vi "Reference Generation.vi"(8 "error in (no error)":errorcluster, 11 "VI in":refnum<vi>) -> (0 "error out":errorcluster, 3 "User Events Reference":refnum<event-registration>)   [LabVIEW 2014, in "User Module.lvlib"]
uses:
  User Module.lvlib
  User Event/User Event Action.ctl
  Queue FGV.ctl
  Message.ctl
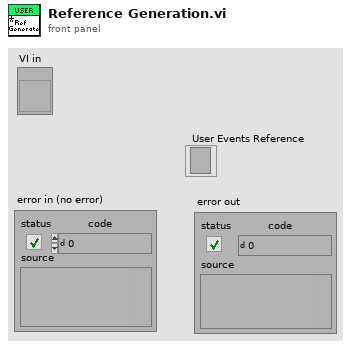
[diagram p1: front panel]
types:
  T1 = typedef "User Module.lvlib/Message.ctl" = cluster{"Message":enum16{"Initialise", "Error", "Close"}, "Data":variant}
  T2 = typedef "User Module.lvlib/Queue FGV.ctl" = enum16{"Set", "Get", "Release"}
  T3 = typedef "User Event Action.ctl" = enum16{"Get", "Create", "Destroy"}
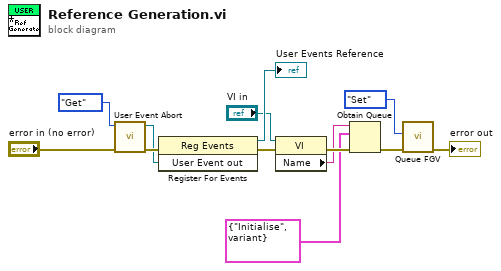
[diagram p0: block diagram]
diagram:
  n1 = call "User Event Abort.vi"("error in (no error)"="error in (no error)", "Action"=User_Event_Action."Get") -> ("error out"=w5:errorcluster, "User Event out"=w4:refnum<user-event>)  [unwired: 8 in]
  n2 = register-events(error in=w5, w4) -> (reference out=→"User Events Reference":refnum<event-registration>, error out=w12:errorcluster)  [unwired: 1 in]
  n3 = property class="VI"(reference="VI in", error in=w12) -> (error out=w8:errorcluster, "Name"=w7:string)  [unwired: 1 out]
  n4 = Obtain Queue(name (unnamed)=w7, element data type=T1 {"Message"=enum."Initialise", "Data"=variant} ("output cluster"), error in (no error)=w8) -> (error out=w9:errorcluster)  [unwired: 2 in, 2 out]
  n5 = call "Queue FGV.vi"("error in (no error)"=w9, "Action"=Queue_FGV."Set") -> ("error out"=→"error out":errorcluster)  [unwired: 8 in, 1 out]
